vi "质控中断报警全局.vi"() -> ()   [LabVIEW 2016, in "质控单元.lvlib"]
panel:
  out "总氮传感器状态显示":bool
  out "总氮超时报警":bool
  out "CODCr传感器状态显示":bool
  out "CODMn传感器状态显示":bool
  out "总磷传感器状态显示":bool
  out "氨氮传感器状态显示":bool
  out "CODCr超时报警":bool
  out "CODMn超时报警":bool
  out "总磷超时报警":bool
  out "氨氮进样超时报警":bool
  out "CODCr中断报警":bool
  out "CODMn中断报警":bool
  out "总氮中断报警":bool
  out "总磷中断报警":bool
  out "氨氮中断报警":bool
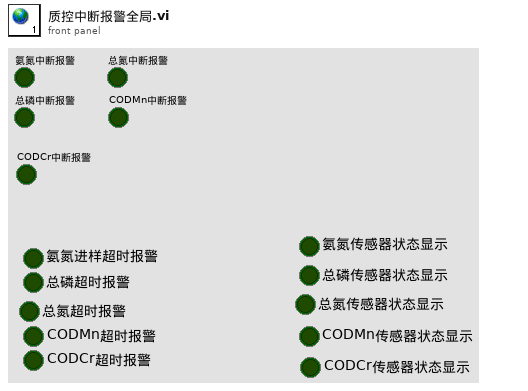
[diagram p1: front panel]
diagram:
